vi "Set focus.vi"(8 "error in (no error)":errorcluster, 10 "Control ref":refnum<vi>, 11 "DatagridElement in":refnum<class "DatagridElement.lvclass">) -> (0 "error out":errorcluster, 2 "Control out":refnum<vi>, 3 "DatagridElement out":refnum<class "DatagridElement.lvclass">)   [LabVIEW 2018, in "D Datagrid Library.lvlib" / "DatagridElement.lvclass"]
doc: "This VI is called to set the proper focus on the control. Most controls will, by default, use the parent implementation, which just sets the keyfocus property. Some controls may need different implementations. Those should override this VI."
uses:
  DatagridElement.lvclass
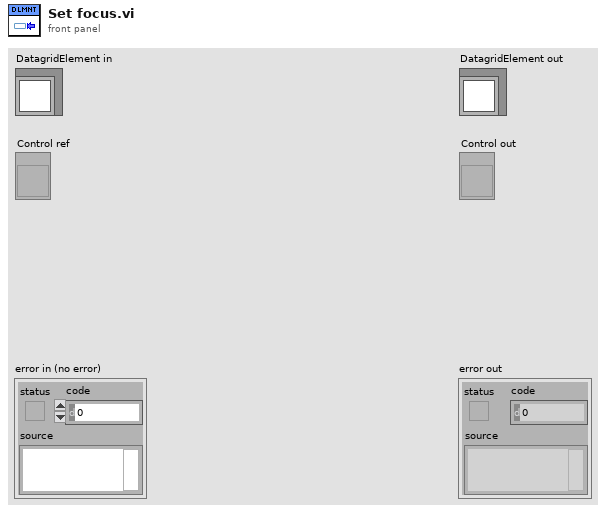
[diagram p1: front panel]
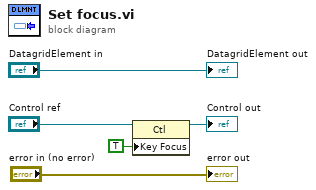
[diagram p0: block diagram]
diagram:
  n1 = property class="Ctl"(reference="Control ref", "Key Focus"=TRUE) -> (reference out=→"Control out":refnum<vi>)  [unwired: 1 in, 1 out]
  "error out" <- "error in (no error)"
  "DatagridElement out" <- "DatagridElement in"
